vi "Check Log Size.vi"(8 "error in":errorcluster, 11 "Log Producer in":refnum<class "Log Producer.lvclass">) -> (0 "error out":errorcluster, 1 "current filename":path, 2 "log in progress":bool, 3 "Log Producer out":refnum<class "Log Producer.lvclass">)   [LabVIEW 2020, in "Log Producer.lvclass"]
uses:
  Log Producer.lvclass
  Log Producer.lvclass/Log Producer.ctl
  Logger Interface/Logger Interface.lvclass
  Frame Logging.lvlib
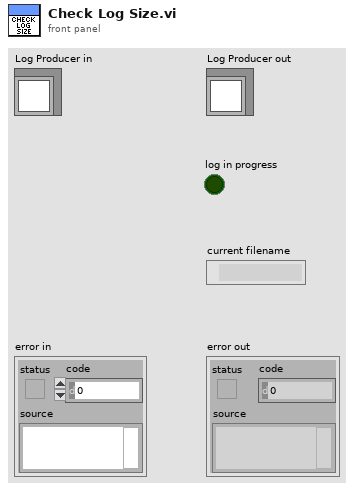
[diagram p1: front panel]
types:
  T1 = typedef "AIM ARINC 664 Engine.lvlib/Implementation.lvlib/Frame Logging.lvlib/Logger Data Reference.ctl" = refnum<data-value>
  T2 = typedef "loggingThreshold_types.ctl" = cluster{"segmentation threshold":dbl, "DiskSpaceThPerc":dbl, "checkDiskSpace":bool, "segmentFiles":bool, "Segment Files By":u16}
  T3 = cluster{"Logger Interface.lvclass":refnum<class "Logger Interface.lvclass">}
  T4 = enum16{"no action", "close file", "segment file"}
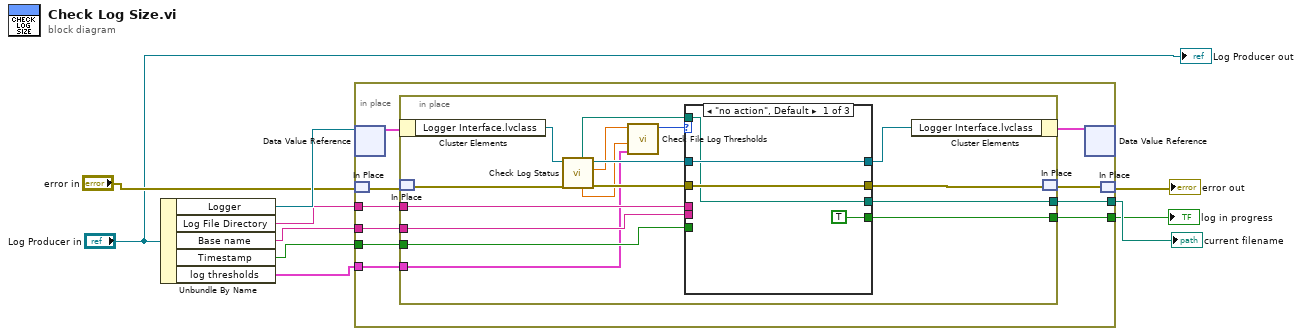
[diagram p0: block diagram]
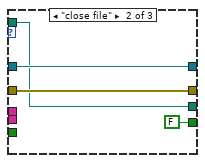
[diagram p2: hidden frame]
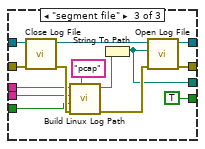
[diagram p3: hidden frame]
diagram:
  n1 = Unbundle By Name("Log Producer in") -> ("Logger"=w10:T1, "Log File Directory"=w8:string, "Base name"=w7:string, "Timestamp"=w6:bool, "log thresholds"=w5:T2)
  n2 = in-place {
    in-place-border: w8 -> [w16]
    in-place-border: w7 -> [w15]
    in-place-border: w6 -> [w14]
    in-place-border: [w13] -> w2
    in-place-border: [w12] -> w1
    in-place-border: w5 -> [w11]
    n3 = in-place-dvr #1(w10) -> (w20:T3)  [unwired: 1 out]
    n4 = in-place-match #2("error in") -> (w19:errorcluster)
    n5 = in-place {
      in-place-border: w16 -> [w31]
      in-place-border: w15 -> [w30]
      in-place-border: w14 -> [w29]
      in-place-border: [w28] -> w13
      in-place-border: [w23] -> w12
      in-place-border: w11 -> [w21]
      n6 = in-place-cluster #3(w20) -> ("Logger Interface.lvclass"=w36:refnum<class "Logger Interface.lvclass">)
      n7 = in-place-match #4(w19) -> (w35:errorcluster)
      n8 = call-dynamic "Check Log Status.vi"("error in"=w35, "Logger Interface in"=w36) -> ("error out"=w27:errorcluster, "Log file Size MB"=w26:dbl, "Logger Interface out"=w33:refnum<class "Logger Interface.lvclass">, "Hard Drive Space Used (%)"=w25:dbl, "current filename"=w22:path)  [unwired: 5 in]
      n9 = call "Check File Log Thresholds.vi"("log thresholds"=w21, "Hard Drive Space Used (%)"=w25, "Log file Size MB"=w26) -> ("action"=w24:T4)  [unwired: 8 in]
      n10 = case shown="\"no action\", Default" w24 {
        tunnel: w33 -> [w40 w44 w58]
        tunnel: w27 -> [w39 w43 w56]
        tunnel: [w39 w43 w55] -> w32
        tunnel: [w40 w44 w54] -> w34
        tunnel: w31 -> [_ _ w49]
        tunnel: w30 -> [_ _ w48]
        tunnel: w29 -> [_ _ w47]
        tunnel: [w37 w41 w46] -> w28
        tunnel: [TRUE ("log in progress") FALSE ("log in progress") TRUE ("log in progress")] -> w23
        tunnel: w22 -> [w37 w41 _]
        frame "no action", Default {
        }
        frame "close file" {
        }
        frame "segment file" {
          n11 = call-dynamic "Close Log File.vi"("error in (no error)"=w56, "Logger Interface in"=w58) -> ("error out"=w52:errorcluster, "Logger Interface out"=w57:refnum<class "Logger Interface.lvclass">)  [unwired: 8 in]
          n12 = call "Build Linux Log Path.vi"("Extension"="pcap", "error in (no error)"=w52, "Timestamp"=w47, "Name"=w48, "Log File Directory"=w49) -> ("error out"=w51:errorcluster, "Log File Path"=w50:string)  [unwired: 5 in]
          n13 = String To Path(string=w50) -> (path=w46:path)
          n14 = call-dynamic "Open Log File.vi"("error in (no error)"=w51, "Path"=w46, "Logger Interface in"=w57) -> ("error out"=w55:errorcluster, "Logger Interface out"=w54:refnum<class "Logger Interface.lvclass">)  [unwired: 7 in]
        }
      }
      n15 = in-place-cluster #3("Logger Interface.lvclass"=w34) -> (w18:T3)
      n16 = in-place-match #4(w32) -> (w17:errorcluster)
    }
    n17 = in-place-dvr #1(w18) -> ()  [unwired: 2 out]
    n18 = in-place-match #2(w17) -> (→"error out":errorcluster)
  }
  "log in progress" <- w1
  "current filename" <- w2
  "Log Producer out" <- "Log Producer in"
